vi "Update VS channels (object data).vi"(9 "reflectAttributeValues in":T1, 10 "hla map helpers in":T6, 11 "values in":dbl[](array[numeric])) -> (1 "reflectAttributeValues out":T1, 2 "hla map helpers out":T6, 3 "values out":dbl[](array[numeric]))   [LabVIEW 2019, in "HLA Custom Device Engine.lvlib"]
uses:
  HLA Custom Device Engine.lvlib
  RThlaMapHelpers.ctl
  map_interaction.ctl
  map_interaction_value.ctl
  map_attr_param_data.ctl
  map_object.ctl
  map_object_key.ctl
  map_object_value.ctl
  map_object_instance.ctl
  map_object_instance_value.ctl
  map_object_vs_instance.ctl
  reflectAttributeValues_type.ctl
  object_info_received_type.ctl
  emea-ni-adg-hla-lv/src/library/typedefs/TransportationType.ctl
  emea-ni-adg-hla-lv/src/library/typedefs/OrderType.ctl
  dataElement_type.ctl
  Data Encoding_Decoding/HLA Data Conversion.lvlib
  emea-ni-adg-hla-lv/src/library/openrti_rti1516eLv.lvlib
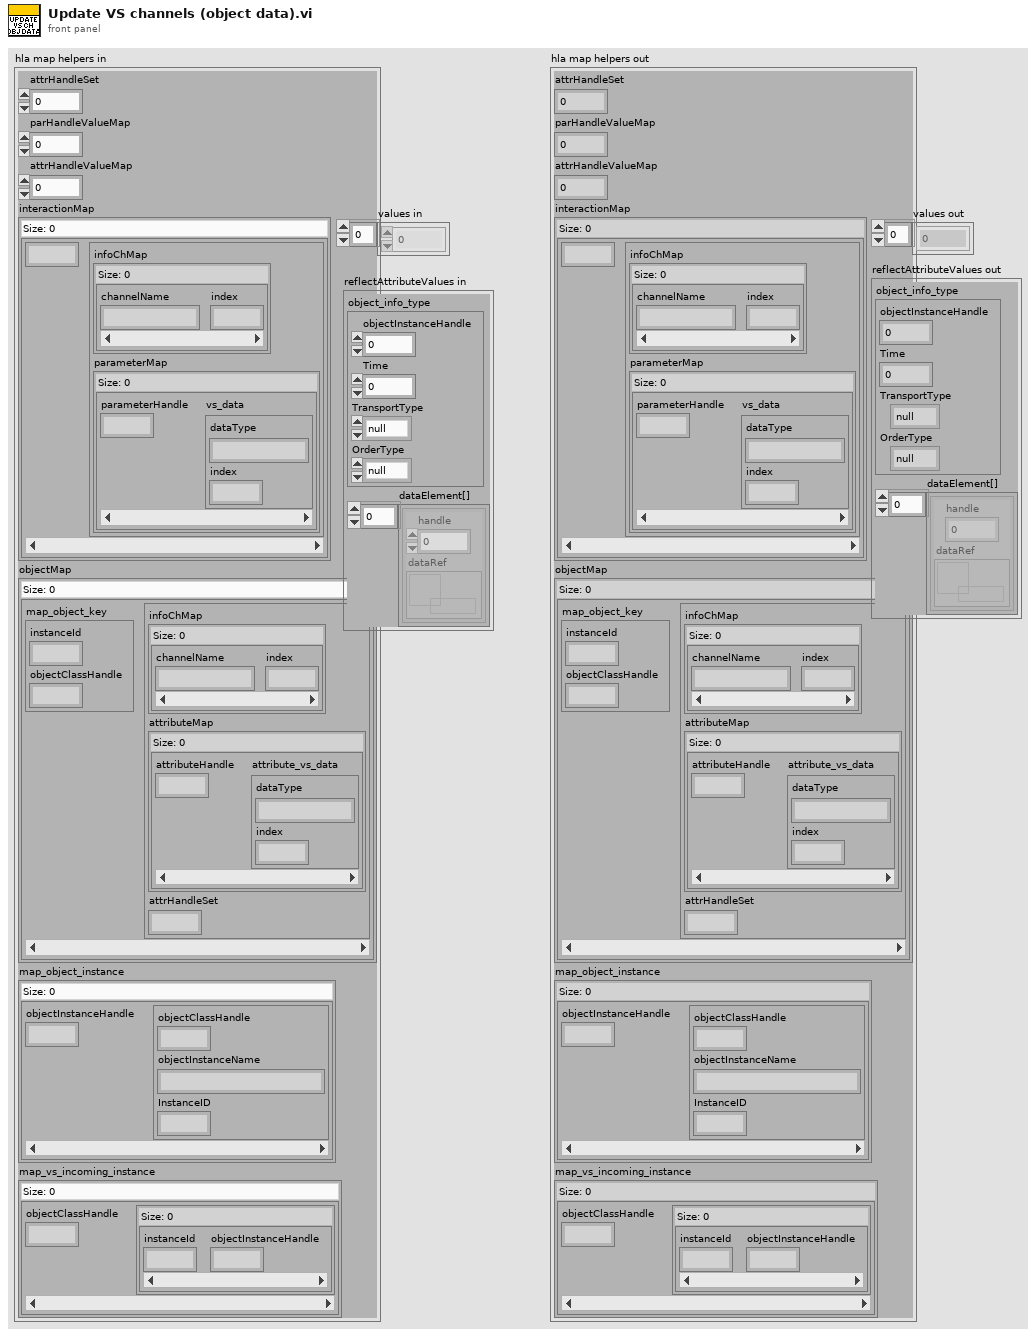
[diagram p1: front panel]
types:
  T1 = typedef "HLA Custom Device Engine.lvlib/reflectAttributeValues_type.ctl" = cluster{"object_info_type":T2, "dataElement[]":T5[]}
  T2 = typedef "HLA Custom Device Engine.lvlib/object_info_received_type.ctl" = cluster{"objectInstanceHandle":u64, "Time":u32, "TransportType":T3, "OrderType":T4}
  T3 = typedef "openrti_rti1516eLv.lvlib/TransportationType.ctl" = enum32{"null", "RELIABLE", "BEST_EFFORT"}
  T4 = typedef "openrti_rti1516eLv.lvlib/OrderType.ctl" = enum32{"null", "RECEIVE", "TIMESTAMP"}
  T5 = typedef "HLA Custom Device Engine.lvlib/dataElement_type.ctl" = cluster{"handle":u64, "dataRef":refnum<data-value>}
  T6 = typedef "RThlaMapHelpers.ctl" = cluster{"attrHandleSet":u64, "parHandleValueMap":u64, "attrHandleValueMap":u64, "interactionMap":T7, "objectMap":T10, "map_object_instance":T13, "map_vs_incoming_instance":T15}
  T7 = typedef "HLA Custom Device Engine.lvlib/map_interaction.ctl" = map{u64, T8}
  T8 = typedef "HLA Custom Device Engine.lvlib/map_interaction_value.ctl" = cluster{"infoChMap":map{string, i32}, "parameterMap":map{u64, T9}}
  T9 = typedef "HLA Custom Device Engine.lvlib/map_attr_param_data.ctl" = cluster{"dataType":string, "index":i32}
  T10 = typedef "HLA Custom Device Engine.lvlib/map_object.ctl" = map{T11, T12}
  T11 = typedef "HLA Custom Device Engine.lvlib/map_object_key.ctl" = cluster{"instanceId":i32, "objectClassHandle":u64}
  T12 = typedef "HLA Custom Device Engine.lvlib/map_object_value.ctl" = cluster{"infoChMap":map{string, i32}, "attributeMap":map{u64, T9}, "attrHandleSet":u64}
  T13 = typedef "HLA Custom Device Engine.lvlib/map_object_instance.ctl" = map{u64, T14}
  T14 = typedef "HLA Custom Device Engine.lvlib/map_object_instance_value.ctl" = cluster{"objectClassHandle":u64, "objectInstanceName":string, "InstanceID":i32}
  T15 = typedef "map_object_vs_instance.ctl" = map{u64, map{i32, u64}}
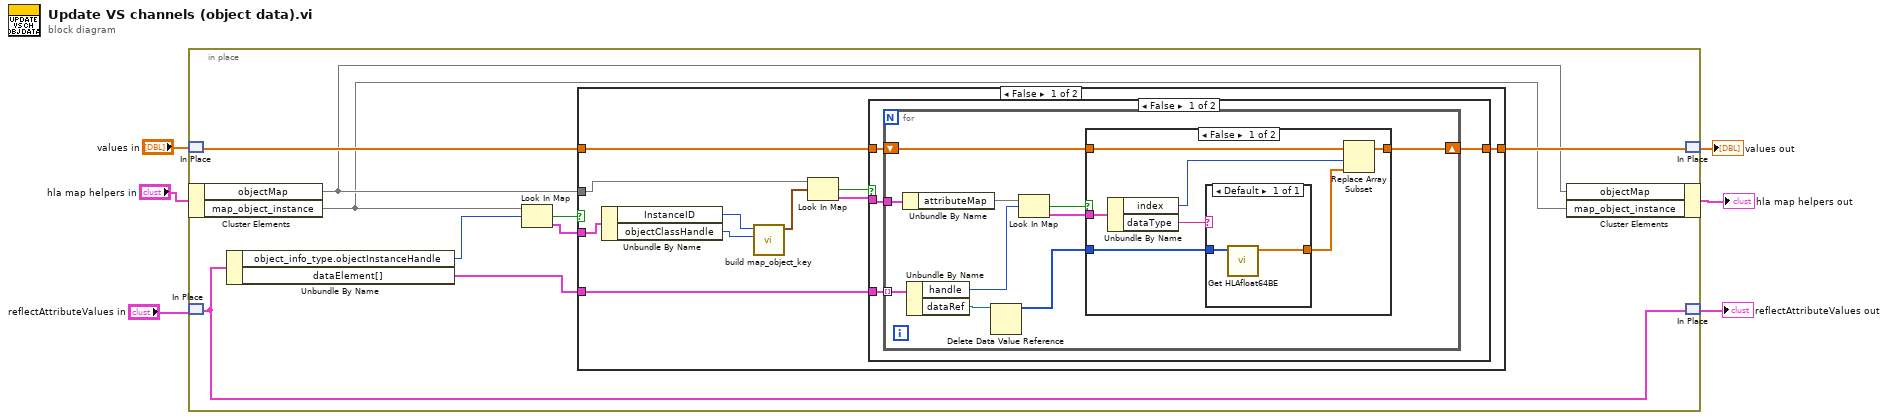
[diagram p0: block diagram]
diagram:
  n1 = in-place {
    n2 = in-place-match #1("values in") -> (w15:dbl[])
    n3 = in-place-cluster #2("hla map helpers in") -> ("objectMap"=w8:T10, "map_object_instance"=w7:T13)
    n4 = in-place-match #3("reflectAttributeValues in") -> (w12:T1)
    n5 = Unbundle By Name(w12) -> ("object_info_type.objectInstanceHandle"=w11:u64, "dataElement[]"=w13:T5[])
    n6 = Look In Map(map=w7, key=w11) -> (key not found?=w10:bool, value=w9:T14)  [unwired: 1 in]
    n7 = case shown="False" w10 {
      tunnel: w15 -> [w23 w51]
      tunnel: [w22 w51] -> w14
      tunnel: w13 -> [w21 _]
      tunnel: w8 -> [w20 _]
      tunnel: w9 -> [w19 _]
      frame False {
        n8 = Unbundle By Name(w19) -> ("InstanceID"=w16:i32, "objectClassHandle"=w18:u64)
        n9 = call "build map_object_key.vi"("objectClassHandle"=w18, "instanceId"=w16) -> ("object_map_key"=w17:T11)  [unwired: 9 in]
        n10 = Look In Map(map=w20, key=w17) -> (key not found?=w25:bool, value=w24:T12)  [unwired: 1 in]
        n11 = case shown="False" w25 {
          tunnel: [w29 w50] -> w22
          tunnel: w24 -> [w28 _]
          tunnel: w23 -> [w27 w50]
          tunnel: w21 -> [w26 _]
          frame False {
            n12 = for {
              tunnel: w28 -> [w32]
              tunnel: w26 -> [w35] mode=indexing
              shift-right: [w38] -> w29
              shift-left: w27 -> [w36]
              n13 = Unbundle By Name(w32) -> ("attributeMap"=w31:map{u64, T9})
              n14 = Unbundle By Name(w35) -> ("handle"=w30:u64, "dataRef"=w34:refnum<data-value>)
              n15 = Delete Data Value Reference(data value reference=w34) -> (data value=w33:u8[])  [unwired: 1 in, 1 out]
              n16 = Look In Map(map=w31, key=w30) -> (key not found?=w39:bool, value=w37:T9)  [unwired: 1 in]
              n17 = case shown="False" w39 {
                tunnel: [w46 w49] -> w38
                tunnel: w37 -> [w42 _]
                tunnel: w36 -> [w44 w49]
                tunnel: w33 -> [w43 _]
                frame False {
                  n18 = Unbundle By Name(w42) -> ("index"=w40:i32, "dataType"=w41:string)
                  n19 = case shown="Default" w41 {
                    tunnel: [w48] -> w45
                    tunnel: w43 -> [w47]
                    frame Default {
                      n20 = call "Get HLAfloat64BE.vi"("raw data in"=w47) -> ("eu data out"=w48:dbl[])  [unwired: 9 in, 1 out]
                    }
                  }
                  n21 = Replace Array Subset(array=w44, new element=w45, index=w40) -> (w46:dbl[])
                }
                frame True {
                }
              }
            }
          }
          frame True {
          }
        }
      }
      frame True {
      }
    }
    n22 = in-place-cluster #2("objectMap"=w8, "map_object_instance"=w7) -> (→"hla map helpers out":T6)
    n23 = in-place-match #1(w14) -> (→"values out":dbl[])
    n24 = in-place-match #3(w12) -> (→"reflectAttributeValues out":T1)
  }
